vi "Measure_Single_Point_With_Compliance.vi"(8 "error in (no error)":errorcluster, 10 "Pin":string, 11 "Keysight_34401A-DMM in":refnum<class "Keysight_34401A-DMM.lvclass">) -> (0 "error out":errorcluster, 2 "DMM_Measurement_Results":T1, 3 "Keysight_34401A-DMM out":refnum<class "Keysight_34401A-DMM.lvclass">)   [LabVIEW 2020, in "Keysight_34401A-DMM.lvclass"]
uses:
  Keysight_34401A-DMM.lvclass
  DMM_Base/Typedef/DMM_Measurement_Results.ctl
  <instrlib>/Agilent 34401/Public/Data/Read (Single Point).vi
  <instrlib>/Agilent 34401/Agilent 34401.lvlib
  DMM_Base/DMM_Base.lvclass
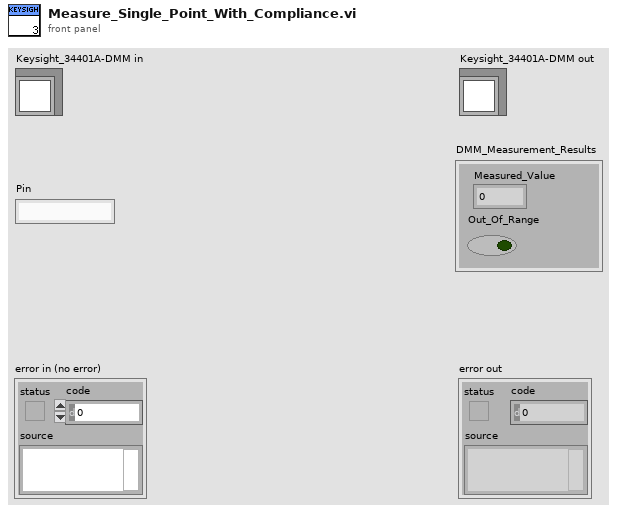
[diagram p1: front panel]
types:
  T1 = typedef "DMM_Base.lvclass/DMM_Measurement_Results.ctl" = cluster{"Measured_Value":dbl, "Out_Of_Range":bool}
  T2 = typedef "Keysight_34401A-DMM.lvclass/Connection with Session.ctl" = cluster{"connection":T3, "session":refnum<visa-resource-name>}
  T3 = typedef "MeasurementLink Session Management V1.lvlib/Session Reservation.lvclass/Connection.ctl" = cluster{"pin or relay name":string, "site":i32, "instrument type id":string, "channel":string}
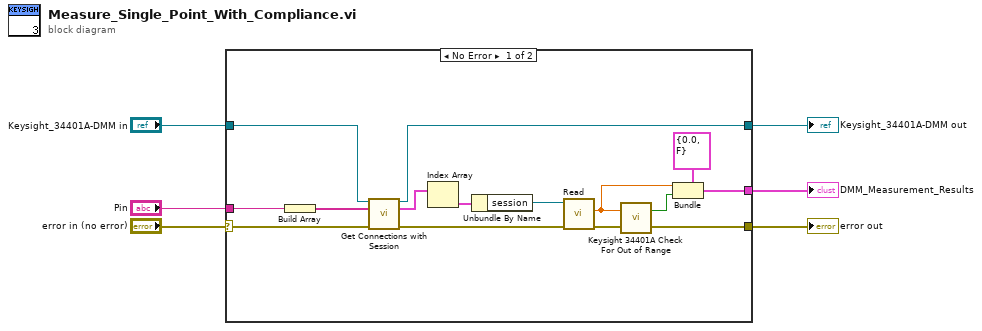
[diagram p0: block diagram]
diagram:
  n1 = case shown="No Error" "error in (no error)" {
    selector: "error in (no error)" -> [w20 w21]
    tunnel: [w19 w21] -> w5
    tunnel: "Keysight_34401A-DMM in" -> [w15 w22]
    tunnel: [w16 w22] -> w2
    tunnel: "Pin" -> [w10 _]
    tunnel: [w9 _] -> w1
    frame No Error {
      n2 = Build Array(w10) -> (w7:string[])
      n3 = call "Get Connections with Session.vi"("Keysight_34401A-DMM in"=w15, "pin or relay names"=w7, "error in (no error)"=w20) -> ("Keysight_34401A-DMM out"=w16:refnum<class "Keysight_34401A-DMM.lvclass">, "connections"=w13:T2[], "error out"=w14:errorcluster)  [unwired: 10 in]
      n4 = Index Array(array=w13) -> (element=w12:T2)  [unwired: 1 in]
      n5 = Unbundle By Name(w12) -> ("session"=w11:refnum<visa-resource-name>)
      n6 = call-poly <instrlib>:"Read.vi"("error in (no error)"=w14, "VISA resource name"=w11) -> ("error out"=w19:errorcluster, "Measurement"=w18:dbl)  [unwired: 7 in, 1 out]
      n7 = call "Keysight 34401A Check For Out of Range.vi"("value"=w18) -> ("out of range?"=w17:bool)  [unwired: 2 in]
      n8 = Bundle(cluster=T1 {"Measured_Value"=0.0, "Out_Of_Range"=FALSE} ("DMM_Measurement_Results"), "Measured_Value"=w18, "Out_Of_Range"=w17) -> (w9:T1)
    }
    frame Error {
    }
  }
  "error out" <- w5
  "Keysight_34401A-DMM out" <- w2
  "DMM_Measurement_Results" <- w1
